vi "Parse Packet Data (Result Set Header).vi"(8 "Error In":errorcluster, 10 "Recieved Bytes":u8[](array[numeric])) -> (0 "Error Out":errorcluster, 2 "Field Count":u64)   [LabVIEW 2014, in "hse-db.lvlib" / "MySQL (TCP).lvlib"]
uses:
  MySQL (TCP).lvlib
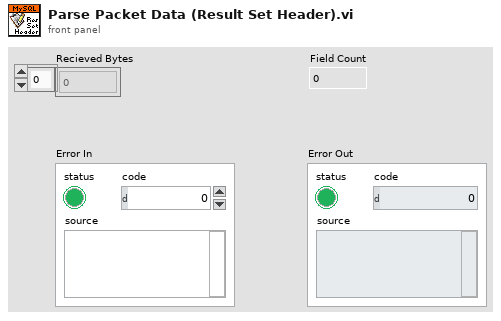
[diagram p1: front panel]
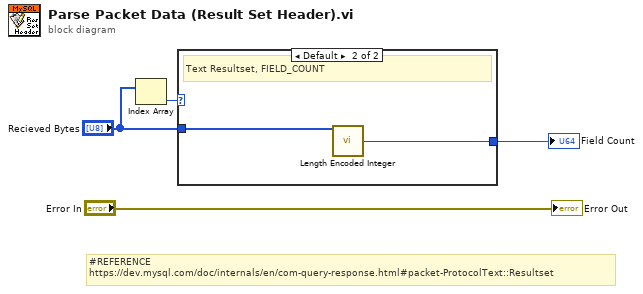
[diagram p0: block diagram]
diagram:
  # "#REFERENCE\nhttps://dev.mysql.com/doc/internals/en/com-query-response.html#packet-ProtocolText::Resultset"
  n1 = Index Array(array="Recieved Bytes") -> (element=w2:u8)  [unwired: 1 in]
  n2 = case shown="Default" w2 {
    tunnel: "Recieved Bytes" -> [_ w6]
    tunnel: [_ w5] -> w1
    frame 251 {
      # "#NOTE\nProtocol::LOCAL_INFILE_Request is not supported and implemented in this toolkit."
      # "LOCAL INFILE Request"
    }
    frame Default {
      # "Text Resultset, FIELD_COUNT"
      n3 = call "Length Encoded Integer.vi"("Bytes in"=w6) -> ("Integer"=w5:u64)  [unwired: 11 in, 3 out]
    }
  }
  "Field Count" <- w1
  "Error Out" <- "Error In"
